vi "File View SubVI.vi"(0 "Channel 8":refnum<vi>, 1 "Channel 1":refnum<vi>, 2 "Config Path":refnum<vi>, 3 "Config file view":bool, 5 "Channel 7":refnum<vi>, 7 "Channel 2":refnum<vi>, 9 "Channel 3":refnum<vi>, 12 "Channel 4":refnum<vi>, 13 "Channel 5":refnum<vi>, 14 "Channel 6":refnum<vi>) -> (4 "File Name":string)   [LabVIEW 2020]
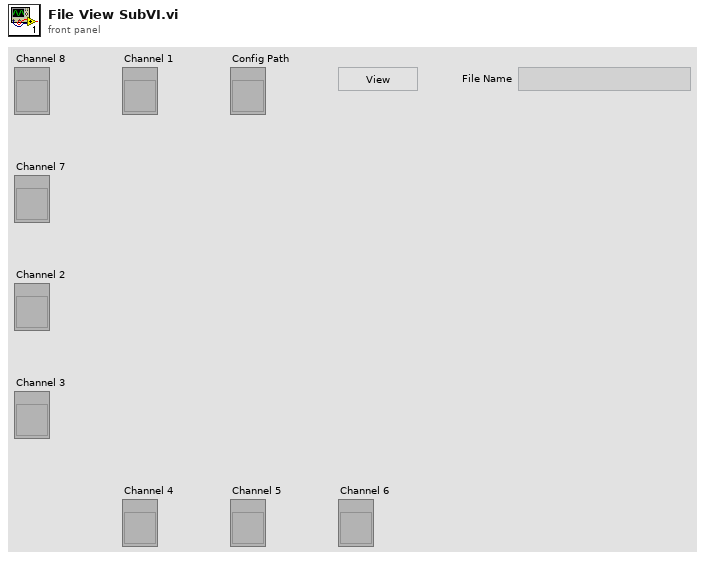
[diagram p1: front panel]
types:
  T1 = cluster{"Port No.":refnum<visa-resource-name>, "Checkbox":bool, "Parity":u16, "Stop Bit":u16, "Baud Rate":dbl, "Data Bits":dbl}[]
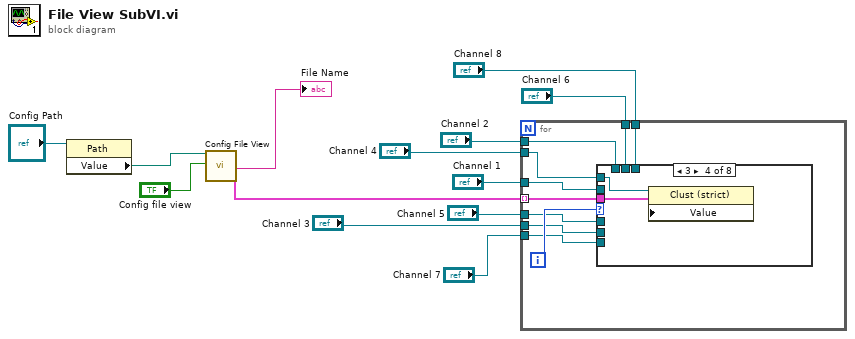
[diagram p0: block diagram]
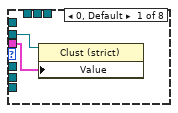
[diagram p2: hidden frame]
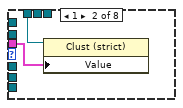
[diagram p3: hidden frame]
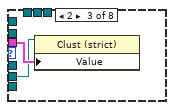
[diagram p4: hidden frame]
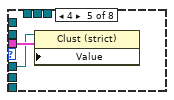
[diagram p5: hidden frame]
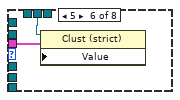
[diagram p6: hidden frame]
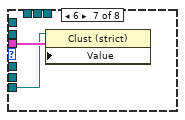
[diagram p7: hidden frame]
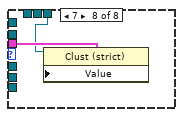
[diagram p8: hidden frame]
diagram:
  n1 = property class="Path"(reference="Config Path") -> ("Value"=w11:path)  [unwired: 1 in, 2 out]
  n2 = call "Config File View.vi"("Path"=w11, "File View"="Config file view") -> ("concatenated string"=→"File Name":string, "data"=w12:T1)  [unwired: 16 in]
  n3 = for {
    tunnel: w12 -> [w22] mode=indexing
    tunnel: "Channel 1" -> [w21]
    tunnel: "Channel 2" -> [w20]
    tunnel: "Channel 3" -> [w19]
    tunnel: "Channel 4" -> [w18]
    tunnel: "Channel 5" -> [w17]
    tunnel: "Channel 6" -> [w16]
    tunnel: "Channel 7" -> [w15]
    tunnel: "Channel 8" -> [w14]
    i -> [w23]
    n4 = case shown="3" w23 {
      tunnel: w22 -> [w25 w27 w29 w31 w33 w35 w37 w39]
      tunnel: w21 -> [w24 _ _ _ _ _ _ _]
      tunnel: w20 -> [_ w26 _ _ _ _ _ _]
      tunnel: w19 -> [_ _ w28 _ _ _ _ _]
      tunnel: w18 -> [_ _ _ w30 _ _ _ _]
      tunnel: w17 -> [_ _ _ _ w32 _ _ _]
      tunnel: w16 -> [_ _ _ _ _ w34 _ _]
      tunnel: w15 -> [_ _ _ _ _ _ w36 _]
      tunnel: w14 -> [_ _ _ _ _ _ _ w38]
      frame 0, Default {
        n5 = property class="Clust (strict)"(reference=w24, "Value"=w25) -> ()  [unwired: 1 in, 2 out]
      }
      frame 1 {
        n6 = property class="Clust (strict)"(reference=w26, "Value"=w27) -> ()  [unwired: 1 in, 2 out]
      }
      frame 2 {
        n7 = property class="Clust (strict)"(reference=w28, "Value"=w29) -> ()  [unwired: 1 in, 2 out]
      }
      frame 3 {
        n8 = property class="Clust (strict)"(reference=w30, "Value"=w31) -> ()  [unwired: 1 in, 2 out]
      }
      frame 4 {
        n9 = property class="Clust (strict)"(reference=w32, "Value"=w33) -> ()  [unwired: 1 in, 2 out]
      }
      frame 5 {
        n10 = property class="Clust (strict)"(reference=w34, "Value"=w35) -> ()  [unwired: 1 in, 2 out]
      }
      frame 6 {
        n11 = property class="Clust (strict)"(reference=w36, "Value"=w37) -> ()  [unwired: 1 in, 2 out]
      }
      frame 7 {
        n12 = property class="Clust (strict)"(reference=w38, "Value"=w39) -> ()  [unwired: 1 in, 2 out]
      }
    }
  }
